vi "global——result.vi"(8 "all data  2":cluster{i32[], "result":T1}[][](array[cluster]) {"result"."RefCoordsys输出"."Measurement System"."Axis Reference" items=["Direct", "Indirect"]; "result"."RefCoordsys输出"."Measurement System"."Angle (deg)" format="%.2f"; "result"."RefCoordsys输出"."Measurement System"."Origin"."Y" format="%.2f"; "result"."RefCoordsys输出"."Measurement System"."Origin"."X" format="%.2f"; "result"."RefCoordsys输出"."Reference System"."Axis Reference" items=["Direct", "Indirect"]; "result"."RefCoordsys输出"."Reference System"."Angle (deg)" format="%.2f"; "result"."RefCoordsys输出"."Reference System"."Origin"."Y" format="%.2f"; "result"."RefCoordsys输出"."Reference System"."Origin"."X" format="%.2f"}, 10 "all result 2":bool[](array[boolean]), 11 "操作":enum16{"read", "write"}(ring)) -> (0 "all data":cluster{i32[], "result":T1}[][](array[cluster]) {"result"."RefCoordsys输出"."Measurement System"."Axis Reference" items=["Direct", "Indirect"]; "result"."RefCoordsys输出"."Measurement System"."Angle (deg)" format="%.2f"; "result"."RefCoordsys输出"."Measurement System"."Origin"."Y" format="%.2f"; "result"."RefCoordsys输出"."Measurement System"."Origin"."X" format="%.2f"; "result"."RefCoordsys输出"."Reference System"."Axis Reference" items=["Direct", "Indirect"]; "result"."RefCoordsys输出"."Reference System"."Angle (deg)" format="%.2f"; "result"."RefCoordsys输出"."Reference System"."Origin"."Y" format="%.2f"; "result"."RefCoordsys输出"."Reference System"."Origin"."X" format="%.2f"}, 2 "all result":bool[](array[boolean]))   [LabVIEW 2015]
uses:
  aoiresultOUT.ctl
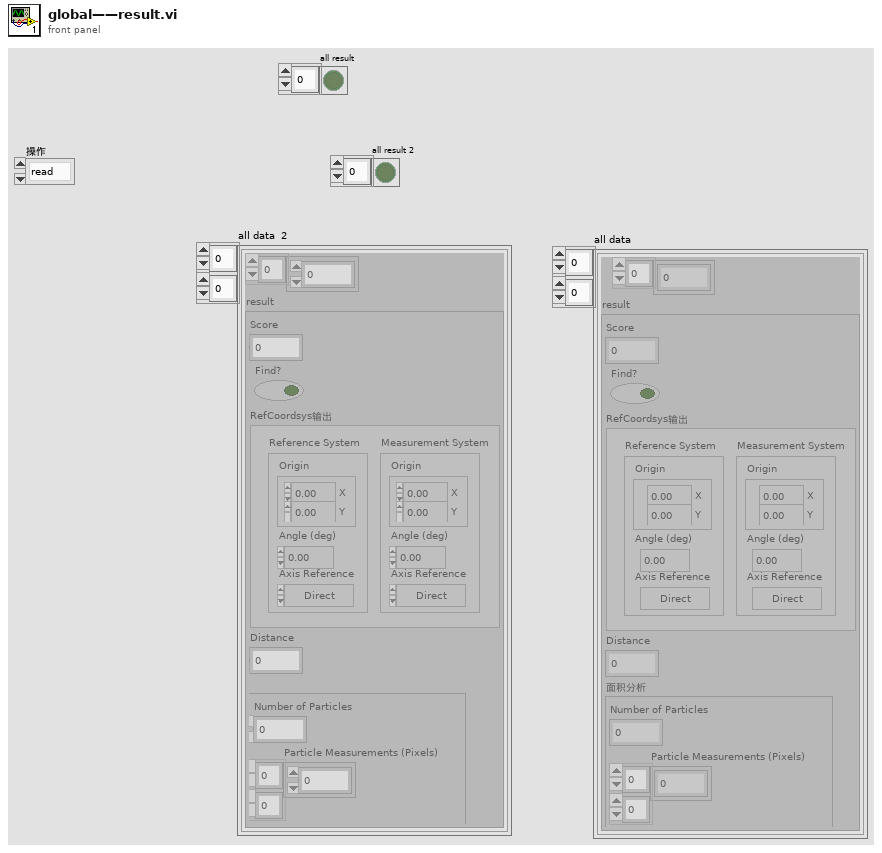
[diagram p1: front panel]
types:
  T1 = typedef "aoiresultOUT.ctl" = cluster{"Score":sgl, "Find?":bool, "RefCoordsys输出":T2, "Distance":sgl, "面积分析":cluster{"Number of Particles":i32, "Particle Measurements (Pixels)":dbl[][]}}
  T2 = typedef "IMAQ Coordinate System" = cluster{"Reference System":cluster{"Origin":cluster{"X":sgl, "Y":sgl}, "Angle (deg)":sgl, "Axis Reference":u32}, "Measurement System":cluster{"Origin":cluster{"X":sgl, "Y":sgl}, "Angle (deg)":sgl, "Axis Reference":u32}}
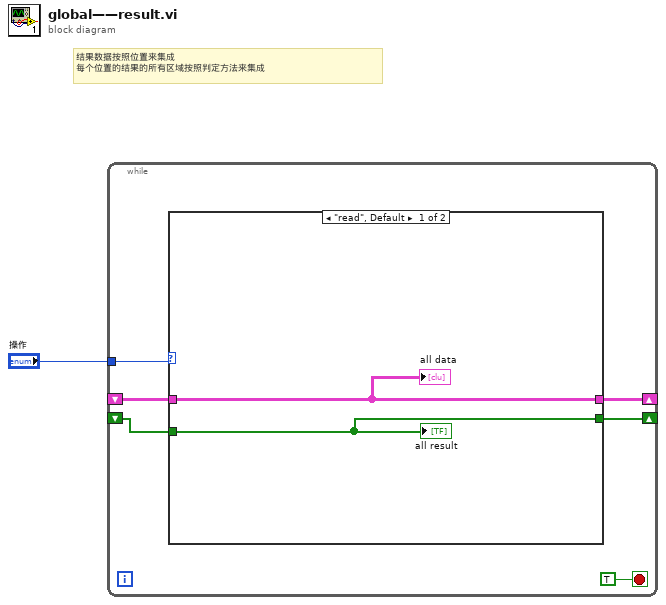
[diagram p0: block diagram]
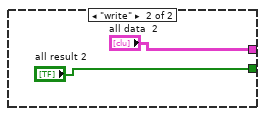
[diagram p2: hidden frame]
diagram:
  # "结果数据按照位置来集成\n每个位置的结果的所有区域按照判定方法来集成"
  n1 = while {
    tunnel: "操作" -> [w6]
    shift-right: [w3] -> _
    shift-left: _ -> [w5]
    shift-right: [w2] -> _
    shift-left: _ -> [w4]
    stop <- TRUE stop-if-true
    n2 = case shown="\"read\", Default" w6 {
      tunnel: w5 -> [w9 _]
      tunnel: w4 -> [w8 _]
      tunnel: [w9 "all data  2"] -> w3
      tunnel: [w8 "all result 2"] -> w2
      frame "read", Default {
        "all data" <- w9
        "all result" <- w8
      }
      frame "write" {
      }
    }
  }
